vi "ObtainQueue.vi"(0 "Queue Names":string[](array[string]), 1 "max queue size (-1, unlimited)":i32=-1, 11 "error in (no error)":errorcluster, 12 "Queue Name Index":i32) -> (4 "MessageQueue":refnum<queue>, 15 "error out":errorcluster)   [LabVIEW 2018, in "AcPwrPlugins.lvlib"]
doc: "This VI creates a named queue."
uses:
  AcPwrPlugins.lvlib
  clMessage.ctl
  AcPwrBaseClass/AcPwrBase.lvclass
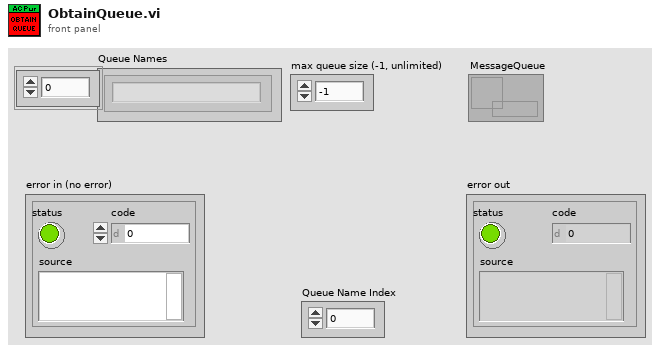
[diagram p1: front panel]
types:
  T1 = typedef "AcPwrPlugins.lvlib/clMessage.ctl" = cluster{"Message":string, "Message Data":variant, "AcPwrBase":refnum<class "AcPwrBase.lvclass">}
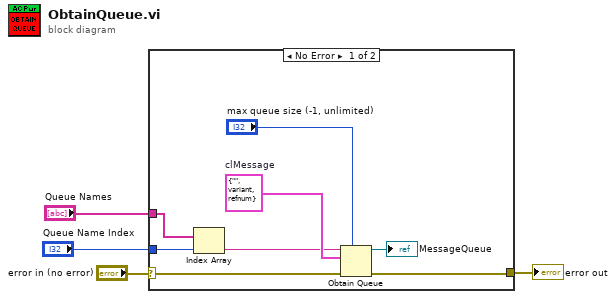
[diagram p0: block diagram]
diagram:
  n1 = case shown="No Error" "error in (no error)" {
    selector: "error in (no error)" -> [w12 w13]
    tunnel: [w11 w13] -> w3
    tunnel: "Queue Names" -> [w6 _]
    tunnel: "Queue Name Index" -> [w7 _]
    frame No Error {
      w8 = T1 {"Message"="", "Message Data"=variant, "AcPwrBase"=refnum}  # clMessage
      n2 = Index Array(array=w6, index=w7) -> (element=w5:string)
      n3 = Obtain Queue(max queue size (-1, unlimited)="max queue size (-1, unlimited)", name (unnamed)=w5, element data type=w8, error in (no error)=w12) -> (queue out=→"MessageQueue":refnum<queue>, error out=w11:errorcluster)  [unwired: 1 in, 1 out]
    }
    frame Error {
    }
  }
  "error out" <- w3
